vi "Write ASIA Global.vi"(8 "error in (no error)":errorcluster, 10 "ASIA Global":T1, 11 "Pump Number":i32) -> (0 "error out":errorcluster, 3 "Pump Number":i32)   [LabVIEW 2018, in "ASIA Pump.lvlib"]
uses:
  ASIA Pump.lvlib
  ASIA Global Element.ctl
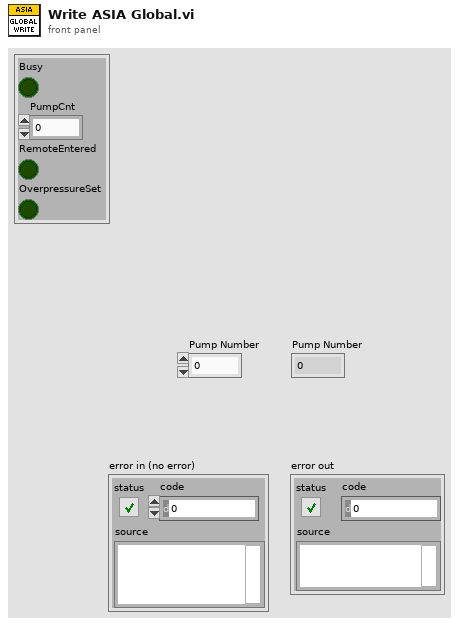
[diagram p1: front panel]
types:
  T1 = typedef "ASIA Pump.lvlib/ASIA Global Element.ctl" = cluster{"Busy":bool, "PumpCnt":dbl, "RemoteEntered":bool, "OverpressureSet":bool}
  T2 = cluster{"Busy":bool, "PumpCnt":dbl, "RemoteEntered":bool, "OverpressureSet":bool}[]
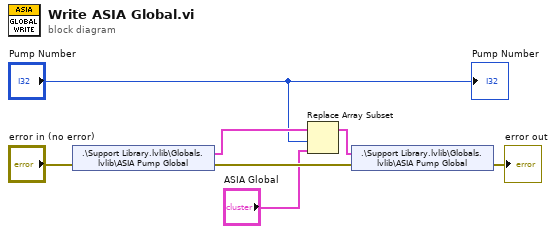
[diagram p0: block diagram]
diagram:
  n1 = shared-variable ".\\Support Library.lvlib\\Globals.lvlib\\ASIA Pump Global"(error in="error in (no error)") -> (w3:T2, error out=w7:errorcluster)
  n2 = Replace Array Subset(array=w3, new element="ASIA Global", index="Pump Number") -> (w4:T2)
  n3 = shared-variable ".\\Support Library.lvlib\\Globals.lvlib\\ASIA Pump Global"(w4, error in=w7) -> (error out=→"error out":errorcluster)
  "Pump Number" <- "Pump Number"
